vi "read_device_object_sdo.vi"(0 "node":u8, 5 "index":u16, 7 "subind":u8, 9 "datasize":u32=128) -> (4 "return":i16, 6 "data":u8[](array[numeric]), 8 "datasize":u32)   [LabVIEW 2011]
uses:
  canopen_dll_master.dll
panel:
  in  "datasize":cluster{"datasize":u32}
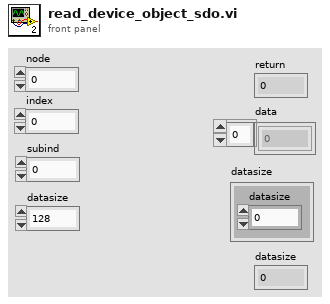
[diagram p1: front panel]
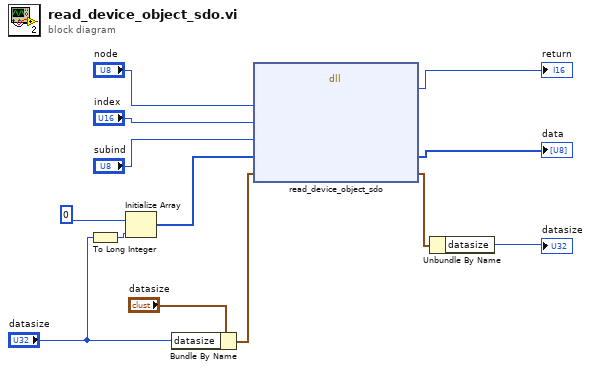
[diagram p0: block diagram]
diagram:
  n1 = To Long Integer(number="datasize") -> (32bit integer=w9:i32)
  n2 = Initialize Array(u8 0 ("data"), w9) -> (w8:u8[])
  n3 = Bundle By Name(cluster="datasize", "datasize"="datasize") -> (w4:cluster{"datasize":u32})
  n4 = dll-call lib="canopen_dll_master.dll" fn="read_device_object_sdo"("node"="node", "index"="index", "subind"="subind", "data"=w8, "datasize"=w4) -> ("return type"=→"return":i16, "data"=→"data":u8[], "datasize"=w3:cluster{"datasize":u32})  [unwired: 6 in, 2 out]
  n5 = Unbundle By Name(w3) -> ("datasize"=→"datasize":u32)
